vi "Open Log File.vi"(8 "error in":errorcluster, 10 "path":path, 11 "CSV word logger in":refnum<class "CSV Word Logger.lvclass">) -> (0 "error out":errorcluster, 3 "CSV word logger out":refnum<class "CSV Word Logger.lvclass">)   [LabVIEW 2020, in "AIM ARINC 429 Engine.lvlib" / "Implementation.lvlib" / "CSV Word Logger.lvclass"]
uses:
  CSV Word Logger.lvclass
  351de733-b961-4ed4-9e08-ca322b6c372e.vi
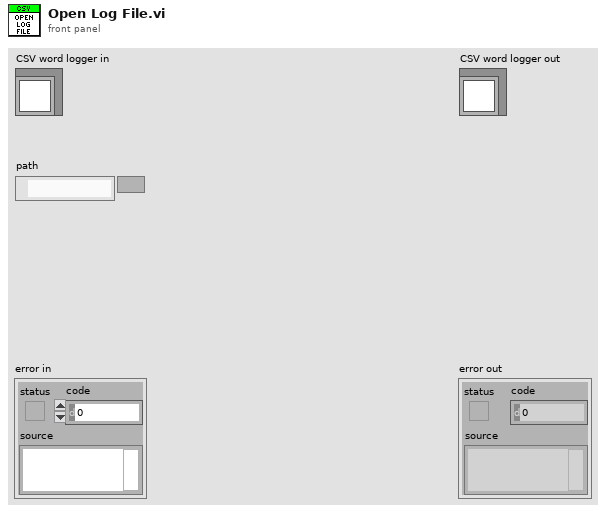
[diagram p1: front panel]
types:
  T1 = enum16{"open", "replace", "create", "open or create", "replace or create", "replace or create with confirmation"}
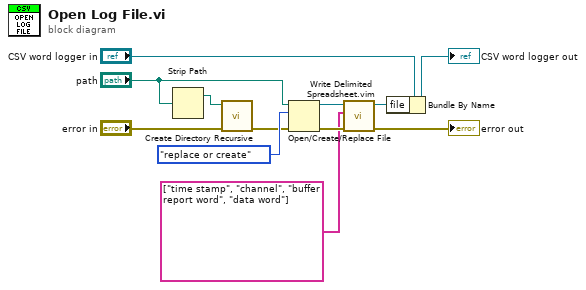
[diagram p0: block diagram]
diagram:
  n1 = Strip Path(path="path") -> (stripped path=w2:path)  [unwired: 1 out]
  n2 = call <vilib>:"Create Directory Recursive.vi"("error in (no error)"="error in", "directory"=w2) -> ("error out"=w4:errorcluster)  [unwired: 3 in, 2 out]
  n3 = Open/Create/Replace File(file path (use dialog)="path", error in=w4, operation (0:open)=T1."replace or create") -> (refnum out=w7:refnum<file>, error out=w9:errorcluster)  [unwired: 3 in, 1 out]
  n4 = call "Write Delimited Spreadsheet.vim"("error in (no error)"=w9, "data"=string[] ["time stamp", "channel", "buffer report word", "data word"], "file in"=w7) -> ("error out"=→"error out":errorcluster, "file out"=w10:refnum<file>)  [unwired: 7 in]
  n5 = Bundle By Name(cluster="CSV word logger in", "file"=w10) -> (→"CSV word logger out":refnum<class "CSV Word Logger.lvclass">)
